vi "Convert Error Cluster to Table.vi"(11 "Error Codes":cluster{i32, string}[](array[cluster])) -> (2 "Code":i32[](array[numeric]), 3 "String":string[](array[string]))   [LabVIEW 2019, in "Ghost Bus Addon System Explorer.lvlib"] (continued)
Explorer</b> window."}, {-307611, "NI VeriStand: The associated NI-XNET database path cannot be found. Please update either the alias or the database path."}, {-307610, "NI VeriStand: The formula contains an invalid function or variable name."}, {-307609, "NI VeriStand: The formula contains an unused variable declaration."}, {-307608, "NI VeriStand: The custom device does not provide a valid source distribution for the target specified. Specify a different target or contact the creator of the custom device for further support."}, {-307607, "NI VeriStand: NI VeriStand could not mutate the system definition file. The system definition file version is different from the official released version of NI VeriStand."}, {-307606, "NI VeriStand: The file does not contain a valid file format."}, {-307605, "NI VeriStand: The requested simulation model could not be found. Navigate to the <b>Model Configuration</b> page in the <b>System Explorer</b> window and choose a different model."}, {-307604, "NI VeriStand: NI VeriStand was unable to mutate the system definition file to the current version."}, {-307603, "NI VeriStand: The requested custom device does not have a main page specified. Contact the creator of the custom device to correct this error."}, {-307602, "NI VeriStand: The GUID could not be found. If the requested page is a custom device, contact the creator of the custom device."}, {-307601, "NI VeriStand: The XML file is invalid according to the XML schema document (XSD)."}, {-307600, "NI VeriStand: The specified VI is broken and cannot run. Open the VI in the LabVIEW development environment for more information."}, {-307562, "NI VeriStand: You cannot use a waveform session reference that you did not first open. Use the NI VeriStand - Open Waveform Session VI to open a waveform session reference."}, {-307561, "NI VeriStand: Cannot write to waveform. Another waveform write session is already open for this waveform reference, and only one writer can access the waveform reference at a time."}, {-307559, "NI VeriStand: The size of an input array does not match the number of waveforms in the streaming session. When you write to a multiple-waveform session, the number of rows in the 2D <B>Data</B> array must match the number of waveforms in the session. When you start a multiple-waveform session, the size of the 1D <B>t0s</B> array must match the number of waveforms in the session."}, {-307557, "NI VeriStand: Custom device cannot perform requested operation because NI VeriStand Engine is shutting down."}, {-307556, "NI VeriStand: Cannot open waveform session because waveform data references are not valid. Use the NI VeriStand - Get Waveform Data Reference VI to generate valid data references with which you can open a waveform session."}, {-307555, "NI VeriStand: Cannot open a waveform session using an empty array of waveform references. Use the NI VeriStand - Get Waveform Data Reference VI to generate valid data references with which you can open a waveform session."}, {-307554, "NI VeriStand: The specified stream condition is not valid for the data type of the waveform. This error might occur if you try to set the streaming condition to be within a range of values for a waveform whose data type is CDB. The in-range streaming condition supports only waveforms whose data type is DBL."}, {-307553, "NI VeriStand: Unexpected waveform data type. This VI requires the specified waveform nodes to be of a specific data type, but the actual data type did not match."}, {-307552, "NI VeriStand: Internal error. An attempt was made to open a 2D waveform read session."}, {-307551, "NI VeriStand: Internal error. The buffered data system failed to find required information in the transaction's variant data."}, {-307550, "NI VeriStand: You have provided an invalid username or password."}, {-307549, "NI VeriStand: Cannot find the wave file that an alarm response is configured to play when the alarm is triggered. Verify that wave files are located at their specified locations. To view and configure this alarm-response setting, open the <B>Project Explorer</B> window, and then double-click an alarm response node underneath <B>Alarm Responses</B> in the tree."}, {-307548, "NI VeriStand: Legacy Stimulus Profile Editor is not supported anymore."}, {-307526, "NI VeriStand: The XML file provided is invalid."}, {-307525, "NI VeriStand: Cannot open selected file. The file was saved in a later version of NI VeriStand."}, {-307512, "NI VeriStand: An unexpected step error has occured."}, {-307511, "NI VeriStand: EESPort with the given name already exists."}, {-307510, "NI VeriStand: Framework with the given name already exists."}, {-307505, "NI VeriStand: The FPGA bitfile has changed since the system definition file was last compiled. Open the system definition file in the <b>System Explorer</b> window and refresh the FPGA configuration file (.fpgaconfig)."}, {-307504, "NI VeriStand: An FPGA argument or parameter is outside the expected range.  This might be a problem with the FPGA configuration file (.fpgaconfig)."}, {-307503, "NI VeriStand: An unknown exception occurred while running the NI-FPGA device. Verify that NI-RIO and the NI VeriStand software are installed correctly on the real-time (RT) target."}, {-307502, "NI VeriStand: An FPGA argument or parameter is invalid. This might be a problem with the FPGA configuration file (.fpgaconfig) or FPGA bitfile. This problem also might be caused by an invalid FPGA target handle."}, {-307501, "NI VeriStand: The specified operation is unable to acquire the memory necessary to execute. To correct this error, increase the amount of memory in the system or reduce the amount of memory that this operation requires. You can reduce the amount of memory required by the operation by uninstalling unneeded components from the real-time (RT) target or by reducing the number of devices, channels, and/or stimulus generators used."}, {307500, "NI VeriStand: The FPGA configuration file (.fpgaconfig) is invalid or contains an error."}, {-1073807360, "VISA:  (Hex 0xBFFF0000) Unknown system error (miscellaneous error)."}, {-1073807346, "VISA:  (Hex 0xBFFF000E) The given session or object reference is invalid."}, {-1073807345, "VISA:  (Hex 0xBFFF000F) Specified type of lock cannot be obtained, or specified operation cannot be performed, because the resource is locked."}, {-1073807344, "VISA:  (Hex 0xBFFF0010) Invalid expression specified for search."}, {-1073807343, "VISA:  (Hex 0xBFFF0011) Insufficient location information or the device or resource is not present in the system."}, {-1073807342, "VISA:  (Hex 0xBFFF0012) Invalid resource reference specified. Parsing error."}, {-1073807341, "VISA:  (Hex 0xBFFF0013) Invalid access mode."}, {-1073807339, "VISA:  (Hex 0xBFFF0015) Timeout expired before operation completed."}, {-1073807338, "VISA:  (Hex 0xBFFF0016) The VISA driver failed to properly close the session or object reference. This might be due to an error freeing internal or OS resources, a failed network connection, or a lower level driver or OS error."}, {-1073807333, "VISA:  (Hex 0xBFFF001B) Specified degree is invalid."}, {-1073807332, "VISA:  (Hex 0xBFFF001C) Specified job identifier is invalid."}, {-1073807331, "VISA:  (Hex 0xBFFF001D) The specified attribute is not defined or supported by the referenced resource."}, {-1073807330, "VISA:  (Hex 0xBFFF001E) The specified state of the attribute is not valid, or is not supported as defined by the resource."}, {-1073807329, "VISA:  (Hex 0xBFFF001F) The specified attribute is read-only."}, {-1073807328, "VISA:  (Hex 0xBFFF0020) The specified type of lock is not supported by this resource."}, {-1073807327, "VISA:  (Hex 0xBFFF0021) The access key to the specified resource is invalid."}, {-1073807322, "VISA:  (Hex 0xBFFF0026) Specified event type is not supported by the resource."}, {-1073807321, "VISA:  (Hex 0xBFFF0027) Invalid mechanism specified."}, {-1073807320, "VISA:  (Hex 0xBFFF0028) A handler was not installed."}, {-1073807319, "VISA:  (Hex 0xBFFF0029) The given handler reference is invalid."}, {-1073807318, "VISA:  (Hex 0xBFFF002A) Specified event context is invalid."}, {-1073807315, "VISA:  (Hex 0xBFFF002D) The event queue for the specified type has overflowed. This is usually due to previous events not having been closed."}, {-1073807313, "VISA:  (Hex 0xBFFF002F) You must be enabled for events of the specified type in order to receive them."}, {-1073807312, "VISA:  (Hex 0xBFFF0030) User abort occurred during transfer."}, {-1073807308, "VISA:  (Hex 0xBFFF0034) Violation of raw write protocol occurred during transfer."}, {-1073807307, "VISA:  (Hex 0xBFFF0035) Violation of raw read protocol occurred during transfer."}, {-1073807306, "VISA:  (Hex 0xBFFF0036) Device reported an output protocol error during transfer."}, {-1073807305, "VISA:  (Hex 0xBFFF0037) Device reported an input protocol error during transfer."}, {-1073807304, "VISA:  (Hex 0xBFFF0038) Bus error occurred during transfer."}, {-1073807303, "VISA:  (Hex 0xBFFF0039) Unable to queue the asynchronous operation because there is already an operation in progress."}, {-1073807302, "VISA:  (Hex 0xBFFF003A) Unable to start operation because setup is invalid (due to attributes being set to an inconsistent state)."}, {-1073807301, "VISA:  (Hex 0xBFFF003B) Unable to queue the asynchronous operation (usually due to the I/O completion event not being enabled or insufficient space in the session's queue)."}, {-1073807300, "VISA:  (Hex 0xBFFF003C) Insufficient system resources to perform necessary memory allocation."}, {-1073807299, "VISA:  (Hex 0xBFFF003D) Invalid buffer mask specified."}, {-1073807298, "VISA:  (Hex 0xBFFF003E) Could not perform operation because of I/O error."}, {-1073807297, "VISA:  (Hex 0xBFFF003F) A format specifier in the format string is invalid."}, {-1073807295, "VISA:  (Hex 0xBFFF0041) A format specifier in the format string is not supported."}, {-1073807294, "VISA:  (Hex 0xBFFF0042) The specified trigger line is currently in use."}, {-1073807293, "VISA:  (Hex 0xBFFF0043) The specified trigger line has not been reserved."}, {-1073807290, "VISA:  (Hex 0xBFFF0046) The specified mode is not supported by this VISA implementation."}, {-1073807286, "VISA:  (Hex 0xBFFF004A) Service request has not been received for the session."}, {-1073807282, "VISA:  (Hex 0xBFFF004E) Invalid address space specified."}, {-1073807279, "VISA:  (Hex 0xBFFF0051) Invalid offset specified."}, {-1073807278, "VISA:  (Hex 0xBFFF0052) Invalid access width specified."}, {-1073807276, "VISA:  (Hex 0xBFFF0054) Specified offset is not accessible from this hardware."}, {-1073807275, "VISA:  (Hex 0xBFFF0055) Cannot support source and destination widths that are different."}, {-1073807273, "VISA:  (Hex 0xBFFF0057) The specified session is not currently mapped."}, {-1073807271, "VISA:  (Hex 0xBFFF0059) A previous response is still pending, causing a multiple query error."}, {-1073807265, "VISA:  (Hex 0xBFFF005F) No listeners condition is detected (both NRFD and NDAC are deasserted)."}, {-1073807264, "VISA:  (Hex 0xBFFF0060) The interface associated with this session is not currently the controller in charge."}, {-1073807263, "VISA:  (Hex 0xBFFF0061) The interface associated with this session is not the system controller."}, {-1073807257, "VISA:  (Hex 0xBFFF0067) The given session or object reference does not support this operation."}, {-1073807256, "VISA:  (Hex 0xBFFF0068) An interrupt is still pending from a previous call."}, {-1073807254, "VISA:  (Hex 0xBFFF006A) A parity error occurred during transfer."}, {-1073807253, "VISA:  (Hex 0xBFFF006B) A framing error occurred during transfer."}, {-1073807252, "VISA:  (Hex 0xBFFF006C) An overrun error occurred during transfer. A character was not read from the hardware before the next character arrived."}, {-1073807250, "VISA:  (Hex 0xBFFF006E) The path from trigSrc to trigDest is not currently mapped."}, {-1073807248, "VISA:  (Hex 0xBFFF0070) The specified offset is not properly aligned for the access width of the operation."}, {-1073807247, "VISA:  (Hex 0xBFFF0071) A specified user buffer is not valid or cannot be accessed for the required size."}, {-1073807246, "VISA:  (Hex 0xBFFF0072) The resource is valid, but VISA cannot currently access it."}, {-1073807242, "VISA:  (Hex 0xBFFF0076) Specified width is not supported by this hardware."}, {-1073807240, "VISA:  (Hex 0xBFFF0078) The value of some parameter (which parameter is not known) is invalid."}, {-1073807239, "VISA:  (Hex 0xBFFF0079) The protocol specified is invalid."}, {-1073807237, "VISA:  (Hex 0xBFFF007B) Invalid size of window specified."}, {-1073807232, "VISA:  (Hex 0xBFFF0080) The specified session currently contains a mapped window."}, {-1073807231, "VISA:  (Hex 0xBFFF0081) The given operation is not implemented."}, {-1073807229, "VISA:  (Hex 0xBFFF0083) Invalid length specified."}, {-1073807215, "VISA:  (Hex 0xBFFF0091) Invalid mode specified."}, {-1073807204, "VISA:  (Hex 0xBFFF009C) The current session did not have a lock on the resource."}, {-1073807203, "VISA:  (Hex 0xBFFF009D) The device does not export any memory."}, {-1073807202, "VISA:  (Hex 0xBFFF009E) VISA or a code library required by VISA could not be located or loaded.  This is usually due to a required driver not being installed on the system."}, {-1073807201, "VISA:  (Hex 0xBFFF009F) The interface cannot generate an interrupt on the requested level or with the requested statusID value."}, {-1073807200, "VISA:  (Hex 0xBFFF00A0) The value specified by the line parameter is invalid."}, {-1073807199, "VISA:  (Hex 0xBFFF00A1) An error occurred while trying to open the specified file. Possible reasons include an invalid path or lack of access rights."}, {-1073807198, "VISA:  (Hex 0xBFFF00A2) An error occurred while performing I/O on the specified file."}, {-1073807197, "VISA:  (Hex 0xBFFF00A3) One of the specified lines, trigSrc or trigDest, is not supported by this VISA implementation, or the combination of lines is not a valid mapping."}, {-1073807196, "VISA:  (Hex 0xBFFF00A4) The specified mechanism is not supported for the given event type."}, {-1073807195, "VISA:  (Hex 0xBFFF00A5) The interface type is valid, but the specified interface number is not configured."}, {-1073807194, "VISA:  (Hex 0xBFFF00A6) The connection for the given session has been lost."}, {-1073807193, "VISA:  (Hex 0xBFFF00A7) The remote machine does not exist or is not accepting any connections. If the NI-VISA server is installed and running on the remote machine, it might have an incompatible version or might be listening on a different port."}, {-1073807192, "VISA:  (Hex 0xBFFF00A8) Access to the resource or remote machine is denied. This is due to lack of sufficient privileges for the current user or machine."}, {-1073807190, "VISA:  (Hex 0xBFFF00AA) A lower level driver reported that this resource corresponds to or is connected to a non-genuine interface. For more information, contact National Instruments support."}, {0, "VISA:  (Hex 0x0) Operation completed successfully."}, {1073676290, "VISA:  (Hex 0x3FFF0002) Specified event is already enabled for at least one of the specified mechanisms."}, {1073676291, "VISA:  (Hex 0x3FFF0003) Specified event is already disabled for at least one of the specified mechanisms."}, {1073676292, "VISA:  (Hex 0x3FFF0004) Operation completed successfully, but queue was already empty."}, {1073676293, "VISA:  (Hex 0x3FFF0005) The specified termination character was read."}, {1073676294, "VISA:  (Hex 0x3FFF0006) The number of bytes transferred is equal to the requested input count. More data might be available."}, {1073676300, "VISA:  (Hex 0x3FFF000C) VISA received more event information of the specified type than the configured queue size could hold."}, {1073676407, "VISA:  (Hex 0x3FFF0077) The specified configuration either does not exist or could not be loaded. VISA-specified defaults will be used."}, {1073676413, "VISA:  (Hex 0x3FFF007D) Session opened successfully, but the device at the specified address is not responding."}, {1073676414, "VISA:  (Hex 0x3FFF007E) The path from trigSrc to trigDest is already mapped."}, {1073676416, "VISA:  (Hex 0x3FFF0080) Wait terminated successfully on receipt of an event notification. There is at least one more event occurrence of the type specified by inEventType available for this session."}, {1073676418, "VISA:  (Hex 0x3FFF0082) The specified object reference is uninitialized."}, {1073676420, "VISA:  (Hex 0x3FFF0084) Although the specified state of the attribute is valid, it is not supported by this resource implementation."}, {1073676421, "VISA:  (Hex 0x3FFF0085) The status code passed to the operation could not be interpreted."}, {1073676424, "VISA:  (Hex 0x3FFF0088) The specified I/O buffer is not supported."}, {1073676440, "VISA:  (Hex 0x3FFF0098) Event handled successfully. Do not invoke any other handlers on this session for this event."}, {1073676441, "VISA:  (Hex 0x3FFF0099) Operation completed successfully, and this session has nested shared locks."}, {1073676442, "VISA:  (Hex 0x3FFF009A) Operation completed successfully, and this session has nested exclusive locks."}, {1073676443, "VISA:  (Hex 0x3FFF009B) Operation completed successfully, but the operation was actually synchronous rather than asynchronous."}, {1073676457, "VISA:  (Hex 0x3FFF00A9) The operation succeeded, but a lower level driver did not implement the extended functionality."}, {-2147483638, "LabVIEW: (Hex 0x8000000A) The data necessary to complete this operation is not yet available."}, {-2147467263, "LabVIEW: (Hex 0x80004001) Not implemented."}, {-2147467262, "LabVIEW: (Hex 0x80004002) No such interface supported."}, {-2147467261, "LabVIEW: (Hex 0x80004003) Invalid pointer."}, {-2147467260, "LabVIEW: (Hex 0x80004004) Operation aborted."}, {-2147467259, "LabVIEW: (Hex 0x80004005) Unspecified error."}, {-2147418113, "LabVIEW: (Hex 0x8000FFFF) Catastrophic failure."}, {-2147024891, "LabVIEW: (Hex 0x80070005) Access denied. This error can occur if you attempt to write a single writer shared variable that is already connected to a subscriber with write access. Ensure that you connect only one target with write access to this shared variable at a time."}, {-2147024890, "LabVIEW: (Hex 0x80070006) Invalid handle."}, {-2147024882, "LabVIEW: (Hex 0x8007000E) Ran out of memory."}, {-2147024809, "LabVIEW: (Hex 0x80070057) One or more arguments are invalid."}, {-2132869120, "LabVIEW: (Hex 0x80DF0000) The assembly you are deploying is bad."}, {-2132869119, "LabVIEW: (Hex 0x80DF0001) The assembly handler does not support the sent command."}, {-2132869118, "LabVIEW: (Hex 0x80DF0002) A file I/O error occurred."}, {-2132869117, "LabVIEW: (Hex 0x80DF0003) The resource you are deploying is bad."}, {-2132869116, "LabVIEW: (Hex 0x80DF0004) The item cannot read the assembly."}, {-2132869115, "LabVIEW: (Hex 0x80DF0005) The item cannot create the assembly handler."}, {-2132869114, "LabVIEW: (Hex 0x80DF0006) A module cannot load."}, {-2132869113, "LabVIEW: (Hex 0x80DF0007) The item encountered an invalid pointer argument."}, {-2132869112, "LabVIEW: (Hex 0x80DF0008) The item cannot be found."}, {-2132869111, "LabVIEW: (Hex 0x80DF0009) The item is out of memory."}, {-2132869110, "LabVIEW: (Hex 0x80DF000A) A communication error between the host and target occurred."}, {-2132869109, "LabVIEW: (Hex 0x80DF000B) The system is in a bad state."}, {-2132869108, "LabVIEW: (Hex 0x80DF000C) The deploy header is bad."}, {-2132869107, "LabVIEW: (Hex 0x80DF000D) An unknown error occurred during deployment."}, {-2132869106, "LabVIEW: (Hex 0x80DF000E) An XML parsing error occurred."}, {-2132869105, "LabVIEW: (Hex 0x80DF000F) The deployment command failed."}, {-2132869104, "LabVIEW: (Hex 0x80DF0010) The current deployment operation has a missing dependency."}, {-2132869103, "LabVIEW: (Hex 0x80DF0011) The item encountered an invalid argument."}, {-2132869102, "LabVIEW: (Hex 0x80DF0012) The specified file cannot be found."}, {-2132869101, "LabVIEW: (Hex 0x80DF0013) The deployment operation caused a rollback operation, and the rollback operation failed."}, {-2132869100, "LabVIEW: (Hex 0x80DF0014) Logging an entry to the rollback log causes an error."}, {-2132869099, "LabVIEW: (Hex 0x80DF0015) A deployment transaction is in progress."}, {-2132869098, "LabVIEW: (Hex 0x80DF0016) A deployment transaction has not started."}, {-2132869096, "LabVIEW: (Hex 0x80DF0018) The deployment operation causes a rollback operation."}, {-2132869095, "LabVIEW: (Hex 0x80DF0019) The deployment connection timed out."}, {-2132869094, "LabVIEW: (Hex 0x80DF001A) The current transaction has no items to process."}, {-2132869093, "LabVIEW: (Hex 0x80DF001B) The current state does not allow the deployment operation."}, {-2132869092, "LabVIEW: (Hex 0x80DF001C) No items are left to deploy."}, {-2132869091, "LabVIEW: (Hex 0x80DF001D) No items are left to undeploy."}, {-2132869090, "LabVIEW: (Hex 0x80DF001E) The deployment plug-in for this item cannot be found. Verify the proper software is installed."}, {-2132869089, "LabVIEW: (Hex 0x80DF001F) An instance of the target-side deployment endpoint already exists."}, {-2132869088, "LabVIEW: (Hex 0x80DF0020) This item cannot upload because another item with the same name exists in the project."}, {-2067353911, "LabVIEW: (Hex 0x84C6AEC9) The data type of a process variable in the EPICS Client I/O server does not match the data type of the corresponding process variable in the IOC."}, {-2067353910, "LabVIEW: (Hex 0x84C6AECA) The connection to the IOC was lost due to a network failure or an IOC error."}, {-2067353909, "LabVIEW: (Hex 0x84C6AECB) The EPICS Server I/O Server cannot be deployed because one or more PV source variables do not exist. Open the configuration dialog to check and correct broken source variables."}, {-2000000013, "LabVIEW: (Hex 0x88CA6BF3) Input Sprockets Failure. The Mac Input Sprockets Toolkit is not properly installed on the machine."}, {-2000000012, "LabVIEW: (Hex 0x88CA6BF4) Close failure. Make sure the device is currently open."}, {-2000000011, "LabVIEW: (Hex 0x88CA6BF5) Read failure. Failed to read the device."}, {-2000000010, "LabVIEW: (Hex 0x88CA6BF6) The device ID being passed in is incorrect. Please connect the device ID parameter from the Initialize VI to the input parameter of the Close Input Device VI."}, {-2000000009, "LabVIEW: (Hex 0x88CA6BF7) The operation cannot be performed while the device is being acquired."}, {-2000000008, "LabVIEW: (Hex 0x88CA6BF8) Invalid device index. Please check to see if the device is attached correctly. Please verify that the device index you passed in to the Initialize Device VI is correct."}, {-2000000007, "LabVIEW: (Hex 0x88CA6BF9) Data is not yet available."}, {-2000000006, "LabVIEW: (Hex 0x88CA6BFA) The operation cannot be performed unless the device is acquired."}, {-2000000005, "LabVIEW: (Hex 0x88CA6BFB) Access to the input device has been lost. You must reacquire access to the input device."}, {-2000000004, "LabVIEW: (Hex 0x88CA6BFC) This object has not been initialized."}, {-2000000003, "LabVIEW: (Hex 0x88CA6BFD) The DirectInput subsystem could not allocate sufficient memory to complete the call. This value is equal to the E_OUTOFMEMORY standard COM return value."}, {-2000000002, "LabVIEW: (Hex 0x88CA6BFE) The application requires a newer version of DirectInput."}, {-2000000001, "LabVIEW: (Hex 0x88CA6BFF) An invalid parameter was passed to the returning function, or the object was not in a state that permitted the function to be called. This value is equal to the E_INVALIDARG standard COM return value."}, {-2000000000, "LabVIEW: (Hex 0x88CA6C00) The application was written for an unsupported prerelease version of DirectInput."}, {-1967390719, "LabVIEW: (Hex 0x8ABC0001) Packet is too short or too long."}, {-1967390717, "LabVIEW: (Hex 0x8ABC0003) Command not allowed in this particular context."}, {-1967390716, "LabVIEW: (Hex 0x8ABC0004) Duplicate item already exists."}, {-1967390715, "LabVIEW: (Hex 0x8ABC0005) Item not found."}, {-1967390714, "LabVIEW: (Hex 0x8ABC0006) Interface object not valid."}, {-1967390713, "LabVIEW: (Hex 0x8ABC0007) Target of Modify() already has an input connection."}, {-1967390712, "LabVIEW: (Hex 0x8ABC0008) Cannot resolve name to a network address."}, {-1967390711, "LabVIEW: (Hex 0x8ABC0009) Network operation timed out."}, {-1967390704, "LabVIEW: (Hex 0x8ABC0010) Socket has been disconnected by its peer."}, {-1967390703, "LabVIEW: (Hex 0x8ABC0011) Could not resolve service to a port address."}, {-1967390702, "LabVIEW: (Hex 0x8ABC0012) Timed out while trying to connect to peer."}, {-1967390701, "LabVIEW: (Hex 0x8ABC0013) Socket startup (WSAStartup) failed."}, {-1967390687, "LabVIEW: (Hex 0x8ABC0021) The URL is to short to contain the minimum amount of information or the pointer is invalid."}, {-1967390686, "LabVIEW: (Hex 0x8ABC0022) Computer name is not present in the URL."}, {-1967390685, "LabVIEW: (Hex 0x8ABC0023) Computer name starts with a non-alphabetic character."}, {-1967390684, "LabVIEW: (Hex 0x8ABC0024) Computer name contains an invalid character."}, {-1967390683, "LabVIEW: (Hex 0x8ABC0025) Process name is not present in the URL."}, {-1967390682, "LabVIEW: (Hex 0x8ABC0026) Process name contains an invalid character."}, {-1967390681, "LabVIEW: (Hex 0x8ABC0027) Point or tag name is not present in the URL."}, {-1967390680, "LabVIEW: (Hex 0x8ABC0028) Point or tag name contains an invalid character."}, {-1967390679, "LabVIEW: (Hex 0x8ABC0029) URL is not properly formatted: not enough '\\' characters at the beginning."}, {-1967390672, "LabVIEW: (Hex 0x8ABC0030) Empty component in point or tag name."}, {-1967390671, "LabVIEW: (Hex 0x8ABC0031) Invalid update rate."}, {-1967390670, "LabVIEW: (Hex 0x8ABC0032) Invalid deadband."}, {-1967390669, "LabVIEW: (Hex 0x8ABC0033) Key conflict for map collection on insert."}, {-1967390668, "LabVIEW: (Hex 0x8ABC0034) Thread initiation failed."}, {-1967390667, "LabVIEW: (Hex 0x8ABC0035) Process manager server is down."}, {-1967390666, "LabVIEW: (Hex 0x8ABC0036) Time stamp at RealTimeTQ not ready."}, {-1967390655, "LabVIEW: (Hex 0x8ABC0041) Object environment server has already shut down."}, {-1967390638, "LabVIEW: (Hex 0x8ABC0052) Item not found."}, {-1967390623, "LabVIEW: (Hex 0x8ABC0061) Attempted to resolve an incomplete URL."}, {-1967390622, "LabVIEW: (Hex 0x8ABC0062) Attempted to resolve an unrecognized URL type."}, {-1967390621, "LabVIEW: (Hex 0x8ABC0063) Process server has already shut down."}, {-1967390620, "LabVIEW: (Hex 0x8ABC0064) Access request denied."}, {-1967390591, "LabVIEW: (Hex 0x8ABC0081) Unable to resolve the host name."}, {-1967390590, "LabVIEW: (Hex 0x8ABC0082) Unable to resolve the IP address returned from gethostbyname()."}, {-1967390575, "LabVIEW: (Hex 0x8ABC0091) Unrecognized attribute name."}, {-1967390574, "LabVIEW: (Hex 0x8ABC0092) Invalid attribute value."}, {-1967390573, "LabVIEW: (Hex 0x8ABC0093) Failed to get or set attribute."}, {-1967390464, "LabVIEW: (Hex 0x8ABC0100) URL does not start with two slashes."}, {-1967390463, "LabVIEW: (Hex 0x8ABC0101) URL starts with more than two slashes."}, {-1967390462, "LabVIEW: (Hex 0x8ABC0102) URL contains two consecutive delimiters."}, {-1967390461, "LabVIEW: (Hex 0x8ABC0103) URL contains a bad machine name."}, {-1967390460, "LabVIEW: (Hex 0x8ABC0104) Unbalanced quotation marks in URL."}, {-1967345152, "LabVIEW: (Hex 0x8ABCB200) Invalid refnum."}, {-1967345151, "LabVIEW: (Hex 0x8ABCB201) Invalid property code."}, {-1967345150, "LabVIEW: (Hex 0x8ABCB202) Invalid privilege ID."}, {-1967345149, "LabVIEW: (Hex 0x8ABCB203) Invalid access type."}, {-1967345148, "LabVIEW: (Hex 0x8ABCB204) Invalid argument."}, {-1967345147, "LabVIEW: (Hex 0x8ABCB205) Entry not found."}, {-1950679041, "LabVIEW: (Hex 0x8BBAFFFF) The prototype of a shared variable whose data type is custom cannot be an empty variant."}, {-1950679040, "LabVIEW: (Hex 0x8BBB0000) The value from this shared variable might not be the most current value from the data source."}, {-1950679039, "LabVIEW: (Hex 0x8BBB0001) Sensor failure"}, {-1950679038, "LabVIEW: (Hex 0x8BBB0002) General device error response."}, {-1950679037, "LabVIEW: (Hex 0x8BBB0003) The shared variable specified in the binding URL does not exist in the process. Ensure that all shared variables are deployed and the variable identifier URL is correct."}, {-1950679036, "LabVIEW: (Hex 0x8BBB0004) General communications failure."}, {-1950679035, "LabVIEW: (Hex 0x8BBB0005) Unable to locate the shared variable in the Shared Variable Engine (SVE). Deployment of this shared variable may have failed, the SVE has not started, or the SVE is too busy to respond to this request."}, {-1950679034, "LabVIEW: (Hex 0x8BBB0006) The shared variable has no value."}, {-1950679033, "LabVIEW: (Hex 0x8BBB0007) The shared variable is inactive."}, {-1950679032, "LabVIEW: (Hex 0x8BBB0008) Sensor inaccurate"}, {-1950679031, "LabVIEW: (Hex 0x8BBB0009) Engineering unit limits exceeded."}, {-1950679030, "LabVIEW: (Hex 0x8BBB000A) Unspecified error"}, {-1950679029, "LabVIEW: (Hex 0x8BBB000B) Math error"}, {-1950679028, "LabVIEW: (Hex 0x8BBB000C) Communications link failure"}, {-1950679027, "LabVIEW: (Hex 0x8BBB000D) NI-PSP has not connected to the server yet"}, {-1950679026, "LabVIEW: (Hex 0x8BBB000E) DNS lookup failed for the server."}, {-1950679025, "LabVIEW: (Hex 0x8BBB000F) The server is not reachable."}, {-1950679024, "LabVIEW: (Hex 0x8BBB0010) Service lookup failed for the server."}, {-1950679023, "LabVIEW: (Hex 0x8BBB0011) The process specified in the binding URL does not exist. Ensure that all shared variables are deployed and the variable identifier URL is correct."}, {-1950679022, "LabVIEW: (Hex 0x8BBB0012) The process was not found or is not responding."}, {-1950679021, "LabVIEW: (Hex 0x8BBB0013) Failed to resolve URL for this shared variable."}, {-1950679020, "LabVIEW: (Hex 0x8BBB0014) Unable to access the shared variable. This error can occur if you attempt to read from a write-only variable or write to a read-only variable, or if you do not have permission to access the variable."}, {-1950679019, "LabVIEW: (Hex 0x8BBB0015) Subscribe failed. This error can occur when a client attempts to connect to a host using Logos, when the host only supports LogosXT."}, {-1950679018, "LabVIEW: (Hex 0x8BBB0016) Invalid URL for this shared variable."}, {-1950679017, "LabVIEW: (Hex 0x8BBB0017) Invalid combination of feature packs"}, {-1950679016, "LabVIEW: (Hex 0x8BBB0018) Invalid float value."}, {-1950679015, "LabVIEW: (Hex 0x8BBB0019) Invalid Boolean value."}, {-1950679014, "LabVIEW: (Hex 0x8BBB001A) Value attribute not found."}, {-1950679013, "LabVIEW: (Hex 0x8BBB001B) Invalid access type."}, {-1950679012, "LabVIEW: (Hex 0x8BBB001C) Missing access type."}, {-1950679011, "LabVIEW: (Hex 0x8BBB001D) Invalid URL syntax."}, {-1950679010, "LabVIEW: (Hex 0x8BBB001E) Shared variable is bound but the path or URL is not specified."}, {-1950679009, "LabVIEW: (Hex 0x8BBB001F) A path and URL are both specified."}, {-1950679008, "LabVIEW: (Hex 0x8BBB0020) Invalid value for the <b>Enable Aliasing</b> option."}, {-1950679007, "LabVIEW: (Hex 0x8BBB0021) A value is missing for the Enable Aliasing option."}, {-1950679006, "LabVIEW: (Hex 0x8BBB0022) Invalid value for Single Writer option."}, {-1950679005, "LabVIEW: (Hex 0x8BBB0023) You must select a name for the shared variable."}, {-1950679004, "LabVIEW: (Hex 0x8BBB0024) Two var type feature packs are selected"}, {-1950679003, "LabVIEW: (Hex 0x8BBB0025) No var type feature pack is selected"}, {-1950679002, "LabVIEW: (Hex 0x8BBB0026) Var type feature packs must be required"}, {-1950679001, "LabVIEW: (Hex 0x8BBB0027) Buffer size must be greater than 1."}, {-1950679000, "LabVIEW: (Hex 0x8BBB0028) Array length must be greater than or equal to 2."}, {-1950678999, "LabVIEW: (Hex 0x8BBB0029) Data points in waveform must be greater than or equal to 1."}, {-1950678998, "LabVIEW: (Hex 0x8BBB002A) Global variables can only be accessed from the local machine."}, {-1950678997, "LabVIEW: (Hex 0x8BBB002B) You cannot use a Variable Node of this type on this target."}, {-1950678996, "LabVIEW: (Hex 0x8BBB002C) The variable configuration is invalid.  Edit the variable properties to correct the configuration."}, {-1950678995, "LabVIEW: (Hex 0x8BBB002D) Variable has undefined data type."}, {-1950678994, "LabVIEW: (Hex 0x8BBB002E) Variable has invalid data type."}, {-1950678993, "LabVIEW: (Hex 0x8BBB002F) The Raw Full Scale value must be greater than the Raw Zero Scale value."}, {-1950678992, "LabVIEW: (Hex 0x8BBB0030) The Raw Scale and/or Engineering Scale is invalid."}, {-1950678991, "LabVIEW: (Hex 0x8BBB0031) The Engineering Full Scale value should not be equal to Engineering Zero Scale value."}, {-1950678990, "LabVIEW: (Hex 0x8BBB0032) Scaling type attribute not specified."}, {-1950678989, "LabVIEW: (Hex 0x8BBB0033) Scaling ranges not fully specified."}, {-1950678988, "LabVIEW: (Hex 0x8BBB0034) The number of arrays, elements, and points per waveform must be greater than or equal to 1."}, {-1950678987, "LabVIEW: (Hex 0x8BBB0035) This piece of configuration does not exist for this type of variable."}, {-1950678986, "LabVIEW: (Hex 0x8BBB0036) Unspecified shared variable error."}, {-1950678985, "LabVIEW: (Hex 0x8BBB0037) Invalid variable name. The name of a variable cannot start with a single quote ('), start or end with a space, or contain a backslash, forward slash, or any of the following backslash '\\' codes: \\r \\n \\t \\b \\s."}, {-1950678984, "LabVIEW: (Hex 0x8BBB0038) Variable names can have a maximum of 255 characters."}, {-1950678983, "LabVIEW: (Hex 0x8BBB0039) The array sizes in the network buffer must be greater than or equal to the array sizes in the real-time FIFO buffer. The waveform sizes in the network buffer must be greater than or equal to the waveform sizes in the real-time FIFO buffer."}, {-1950678982, "LabVIEW: (Hex 0x8BBB003A) The shared variable client-side read buffer is full."}, {-1950678981, "LabVIEW: (Hex 0x8BBB003B) The shared variable client-side read buffer overflowed."}, {-1950678980, "LabVIEW: (Hex 0x8BBB003C) The shared variable server-side write buffer is full."}, {-1950678979, "LabVIEW: (Hex 0x8BBB003D) The shared variable server-side write buffer overflowed."}, {-1950678978, "LabVIEW: (Hex 0x8BBB003E) The project that contains the project library you want to add a shared variable to must be open."}, {-1950678977, "LabVIEW: (Hex 0x8BBB003F) Unable to deploy the library because the name is reserved. You cannot deploy a library named \"System\", \"LV\", or \"FP\". You also cannot deploy a library with a name that starts with \"NI_\"."}, {-1950678976, "LabVIEW: (Hex 0x8BBB0040) Attempted to load, replace, or remove a configuration from a different source. Your configuration might conflict with the NI Scan Engine configuration."}, {-1950678975, "LabVIEW: (Hex 0x8BBB0041) Invalid Integer value."}, {-1950678974, "LabVIEW: (Hex 0x8BBB0042) Invalid Logging String Format"}, {-1950678972, "LabVIEW: (Hex 0x8BBB0044) LabVIEW failed to load Logos."}, {-1950678971, "LabVIEW: (Hex 0x8BBB0045) LabVIEW could not resolve the machine alias for this Shared Variable and is using a cached IP Address instead."}, {-1950678970, "LabVIEW: (Hex 0x8BBB0046) Failed to load rtvarsup, which is required for Shared Variables with the Real-Time FIFO enabled."}, {-1950678969, "LabVIEW: (Hex 0x8BBB0047) Failed to load rtvarnet, which is required for Network-Published Shared Variables with the Real-Time FIFO enabled."}, {-1950678968, "LabVIEW: (Hex 0x8BBB0048) Failed to load nitaglv, which is required for Network-Published Shared Variables."}, {-1950678967, "LabVIEW: (Hex 0x8BBB0049) Aliasee is missing."}, {-1950678966, "LabVIEW: (Hex 0x8BBB004A) Cannot access I/O variables in Direct mode remotely."}, {-1950678965, "LabVIEW: (Hex 0x8BBB004B) The value read is of a data type that cannot be converted to the data type of this Shared Variable node."}, {-1950678964, "LabVIEW: (Hex 0x8BBB004C) Failed to load NI Scan Engine software required for I/O Variable access.  If you are hosting I/O variables on an RT target, ensure that the NI Scan Engine is installed on the RT target. If you are hosting I/O variables on Windows, you must install a Windows I/O driver, such as DeviceNet, that includes NI Scan Engine support. If you are hosting I/O variables in a Windows VI, the VI must be part of an open LabVIEW project. If you are hosting I/O variables in a Windows-built application, the application must be configured to include hardware configuration."}, {-1950678963, "LabVIEW: (Hex 0x8BBB004D) Unable to open the variable connection. A connection to the specified variable is already open using a different data type."}, {-1950678962, "LabVIEW: (Hex 0x8BBB004E) The specified variable does not support the specified read, write, or open operation."}, {-1950678961, "LabVIEW: (Hex 0x8BBB004F) The connection to the variable has been closed."}, {-1950678960, "LabVIEW: (Hex 0x8BBB0050) The specified variable connection is not configured to read timestamps."}, {-1950678959, "LabVIEW: (Hex 0x8BBB0051) The specified I/O Variable is configured with a timeout, but timeouts are not supported when accessing an I/O variable locally."}, {-1950678958, "LabVIEW: (Hex 0x8BBB0052) This property can be called only on an I/O alias."}, {-1950678957, "LabVIEW: (Hex 0x8BBB0053) This property can be called only on an I/O variable."}, {-1950678956, "LabVIEW: (Hex 0x8BBB0054) The property cannot be set when the variable is reserved."}, {-1950678955, "LabVIEW: (Hex 0x8BBB0055) Invalid URL. The URL cannot contain # or ? characters."}, {-1950678954, "LabVIEW: (Hex 0x8BBB0056) The string for the Variable Engine or protocol portion of the URL is invalid."}, {-1950678953, "LabVIEW: (Hex 0x8BBB0057) The URL is invalid."}, {-1950678952, "LabVIEW: (Hex 0x8BBB0058) The URL is invalid.  The URL contains the User Information subcomponent within the Authority which isn't supported by this scheme.  If you included the \"@\" character as part of the Authority and didn't intend for it to signify the User Information field, replace the \"@\" character with its percent encode UTF-8 equivalent form of \"%40\"."}, {-1950678951, "LabVIEW: (Hex 0x8BBB0059) The host name specified in the URL is invalid.  It contains one or more of the characters \":/?#[]@\" which are illegal to use in their decoded form.  If the host name contains one of these characters, replace it with its percent encoded UTF-8 equivalent form.  For example, to specify the host name \"My Machine?\" you must use the string \"My Machine%3F\"."}, {-1950678950, "LabVIEW: (Hex 0x8BBB005A) The port specified in the Authority component of the URL is invalid.  The port must consist of only numeric characters."}, {-1950678949, "LabVIEW: (Hex 0x8BBB005B) The URL contains one or more unsupported path segments.  Path segments of the form \"/./\", \"/../\", and empty path segments \"//\" are not supported."}, {-1950678948, "LabVIEW: (Hex 0x8BBB005C) The path in the URL is invalid."}, {-1950678947, "LabVIEW: (Hex 0x8BBB005D) The specified URL is invalid.  The URL specifies a host name that includes a port.  However, ports are not supported by the specified variable engine."}, {-1950678946, "LabVIEW: (Hex 0x8BBB005E) The specified URL contains a relative path reference, but LabVIEW does not support relative paths in Variable URLs. To correct the problem, use absolute path references instead of relative references. Variable URLs must take one of the following three forms: (1) [Variable Engine]://[Host Name]/[Container Name]/[Variable Name] or (2) //[Host Name]/[Container Name]/[Variable Name] or (3) /[Container Name]/[Variable Name]."}, {-1950678945, "LabVIEW: (Hex 0x8BBB005F) The host name specified in the variable identifier URL does not correspond to the local host, but the specified variable engine URL only supports an operation on the local host. You cannot perform the specified operation on a remotely hosted variable or stream endpoint. Use the PSP Variable Engine URL (ni.var.psp) to read or write a network-published I/O variable or I/O alias remotely."}, {-1950678944, "LabVIEW: (Hex 0x8BBB0060) The Class Identifier property of the variable object specified in the variable identifier URL is incompatible with the refnum configuration. The class of the variable object is not equivalent to or does not derive from the class you configured for the refnum. This error might occur if you try to reference a <b>Variable</b> object, but the specified variable identifier URL does not reference a <b>Variable</b>."}, {-1950678943, "LabVIEW: (Hex 0x8BBB0061) Timed out while attempting to open a connection to the variable."}, {-1950678942, "LabVIEW: (Hex 0x8BBB0062) Scaling coerce attribute not specified."}, {-1950678941, "LabVIEW: (Hex 0x8BBB0063) An empty string is not a valid URL.  If you want to reference the root container within a variable engine, you need to specify the path explicitly using one of the following URL formats: \"[Variable Engine]://[Host Name]\", \"[Variable Engine]:\", or \"/\"."}, {-1950678940, "LabVIEW: (Hex 0x8BBB0064) The remote configuration web service is not installed on the host specified in the URL."}, {-1950678939, "LabVIEW: (Hex 0x8BBB0065) The version of the remote configuration web service installed on the host specified in the URL is not compatible with this version of LabVIEW."}, {-1950678938, "LabVIEW: (Hex 0x8BBB0066) The NI Vision software is not installed.  This datatype can only be used when NI Vision is installed."}, {-1950678937, "LabVIEW: (Hex 0x8BBB0067) An attempt was made to read or write a property that is only valid for readable variable objects."}, {-1950678936, "LabVIEW: (Hex 0x8BBB0068) The specified buffer size is invalid.  Valid values are zero and sizes greater than two.  A buffer size of zero will disable buffering and cause the connection to maintain only the latest value."}, {-1950678935, "LabVIEW: (Hex 0x8BBB0069) The scheme specified in the URL is not supported."}, {-1950678934, "LabVIEW: (Hex 0x8BBB006A) Requires an open variable connection to read or write the specified property."}, {-1074003967, "LabVIEW: (Hex 0xBFFC0001) Parameter 1 is out of range."}, {-1074003966, "LabVIEW: (Hex 0xBFFC0002) Parameter 2 is out of range."}, {-1074003965, "LabVIEW: (Hex 0xBFFC0003) Parameter 3 is out of range."}, {-1074003964, "LabVIEW: (Hex 0xBFFC0004) Parameter 4 is out of range."}, {-1074003963, "LabVIEW: (Hex 0xBFFC0005) Parameter 5 is out of range."}, {-1074003962, "LabVIEW: (Hex 0xBFFC0006) Parameter 6 is out of range."}, {-1074003961, "LabVIEW: (Hex 0xBFFC0007) Parameter 7 is out of range."}, {-1074003960, "LabVIEW: (Hex 0xBFFC0008) Parameter 8 is out of range."}, {-1074003952, "LabVIEW: (Hex 0xBFFC0010) Error interpreting instrument response"}, {-1074003951, "LabVIEW: (Hex 0xBFFC0011) Identification query failed."}, {-1074003950, "LabVIEW: (Hex 0xBFFC0012) Error interpreting the instrument's response."}, {-1074000001, "LabVIEW: (Hex 0xBFFC0F7F) Instrument self-test failure."}, {-1074000000, "LabVIEW: (Hex 0xBFFC0F80) Instrument error query failure."}, {-1073807202, "LabVIEW: (Hex 0xBFFF009E) VISA or a code library required by VISA could not be located or loaded.  This is usually due to a required driver not being installed on the system."}, {-389122, "LabVIEW: (Hex 0xFFFA0FFE) The target device does not have any response. Possible reason: the target device is not present on the network."}, {-389121, "LabVIEW: (Hex 0xFFFA0FFF) The gateway is unable to allocate an internal communication path from the input port to the output port for processing the request. Possible reason: the gateway is either misconfigured or overloaded."}, {-389118, "LabVIEW: (Hex 0xFFFA1002) An extended file area failed to pass a consistency check. You can use the Modbus master to retry the connection, but the Modbus slave may require certain service."}, {-389116, "LabVIEW: (Hex 0xFFFA1004) The Modbus slave is busy. Use the Modbus master to retransmit data at a later time."}, {-389115, "LabVIEW: (Hex 0xFFFA1005) The Modbus slave is processing the request and may spend a long time processing this request."}, {-389114, "LabVIEW: (Hex 0xFFFA1006) An unrecoverable error occurred while the server was attempting to perform the requested action."}, {-389113, "LabVIEW: (Hex 0xFFFA1007) A value contained in the query data field is invalid for the Modbus slave."}, {-389112, "LabVIEW: (Hex 0xFFFA1008) The Modbus slave does not accept the data address contained in the query."}, {-389111, "LabVIEW: (Hex 0xFFFA1009) The Modbus slave does not accept the function code contained in the query."}, {-389107, "LabVIEW: (Hex 0xFFFA100D) The Modbus master does not use a serial protocol and cannot perform the action that you requested. Ensure that you use a serial Modbus master to perform this action."}, {-389106, "LabVIEW: (Hex 0xFFFA100E) The current Modbus slave cannot perform the operation you wanted to perform, because this slave is not a TCP Modbus slave."}, {-389105, "LabVIEW: (Hex 0xFFFA100F) The Modbus slave daemon, also known as background process, failed to launch. Contact National Instruments for technical support."}, {-389104, "LabVIEW: (Hex 0xFFFA1010) The object that you write exceeds 244 bytes in length."}, {-389103, "LabVIEW: (Hex 0xFFFA1011) The object that you specified does not exist in the Modbus slave. Ensure that you specify an object that exists in the Modbus slave. Contact National Instruments for technical support."}, {-389102, "LabVIEW: (Hex 0xFFFA1012) The data that the Modbus slave returned did not match the data that the Modbus master sent for the operation you want to perform. Contact National Instruments for technical support."}, {-389101, "LabVIEW: (Hex 0xFFFA1013) The returned Modbus Encapsulated Interface type was not 0x0E (14). This type is required for the operation you want to perform. Possible reasons: the Modbus slave does not have a device identification; the Modbus slave does not support read operations on its device identification."}, {-389100, "LabVIEW: (Hex 0xFFFA1014) The returned function code does not match the function code in the requested data. Contact National Instruments for technical support."}, {-375800, "LabVIEW: (Hex 0xFFFA4408) You cannot append variable-sized records, such as strings, handles, or arrays, to a datalog file that is larger than 4GB."}, {-375704, "LabVIEW: (Hex 0xFFFA4468) Invalid channel index."}, {-375703, "LabVIEW: (Hex 0xFFFA4469) Data type mismatch."}, {-375702, "LabVIEW: (Hex 0xFFFA446A) Invalid value index."}, {-375701, "LabVIEW: (Hex 0xFFFA446B) The Excel file is not generated by LabVIEW."}, {-375628, "LabVIEW: (Hex 0xFFFA44B4) Invalid ISO3166 code."}, {-375627, "LabVIEW: (Hex 0xFFFA44B5) Invalid transaction."}, {-375626, "LabVIEW: (Hex 0xFFFA44B6) Operation is not permitted because a transaction was not started."}, {-375625, "LabVIEW: (Hex 0xFFFA44B7) Index out of range."}, {-375624, "LabVIEW: (Hex 0xFFFA44B8) Unexpected OS error."}, {-375623, "LabVIEW: (Hex 0xFFFA44B9) The scan operation took too long."}, {-375622, "LabVIEW: (Hex 0xFFFA44BA) WPA communication error."}, {-375621, "LabVIEW: (Hex 0xFFFA44BB) DBus communication error."}, {-375571, "LabVIEW: (Hex 0xFFFA44ED) Unable to complete the current EtherCAT request."}, {-375570, "LabVIEW: (Hex 0xFFFA44EE) Unable to get the current device configuration."}, {-375569, "LabVIEW: (Hex 0xFFFA44EF) Unable to set the primary device."}, {-375568, "LabVIEW: (Hex 0xFFFA44F0) Unable to get a valid dns address."}, {-375567, "LabVIEW: (Hex 0xFFFA44F1) Unable to get valid gateway address."}, {-375566, "LabVIEW: (Hex 0xFFFA44F2) Unable to get valid IP address."}, {-375565, "LabVIEW: (Hex 0xFFFA44F3) Unable to set current IP configuration"}, {-375564, "LabVIEW: (Hex 0xFFFA44F4) Unable to complete current request."}, {-375563, "LabVIEW: (Hex 0xFFFA44F5) Invalid input parameter."}, {-375562, "LabVIEW: (Hex 0xFFFA44F6) The buffer provided was too small."}, {-375561, "LabVIEW: (Hex 0xFFFA44F7) Operation invalid because IP address index is out of range."}, {-375560, "LabVIEW: (Hex 0xFFFA44F8) Operation not permitted because device index is out of range."}, {-375533, "LabVIEW: (Hex 0xFFFA4513) Unable to set option \"Halt on IP failure\"."}, {-375532, "LabVIEW: (Hex 0xFFFA4514) Unable to get the disk space information."}, {-375531, "LabVIEW: (Hex 0xFFFA4515) Unable to get the target's class."}, {-375530, "LabVIEW: (Hex 0xFFFA4516) Unable to get the target's firmware version."}, {-375529, "LabVIEW: (Hex 0xFFFA4517) Unable to get the target's device description."}, {-375528, "LabVIEW: (Hex 0xFFFA4518) Unable to set user comment."}, {-375527, "LabVIEW: (Hex 0xFFFA4519) Unable to get the target's hostname."}, {-375526, "LabVIEW: (Hex 0xFFFA451A) Unable to set the current hostname."}, {-375525, "LabVIEW: (Hex 0xFFFA451B) Unable to get daylight savings rule."}, {-375524, "LabVIEW: (Hex 0xFFFA451C) Unable to set current daylight savings rule."}, {-375523, "LabVIEW: (Hex 0xFFFA451D) Unable to validate the current timezone."}, {-375522, "LabVIEW: (Hex 0xFFFA451E) Unable to get the current timezone."}, {-375521, "LabVIEW: (Hex 0xFFFA451F) Unable to set current timezone."}, {-375520, "LabVIEW: (Hex 0xFFFA4520) Unable to set current language."}, {-375502, "LabVIEW: (Hex 0xFFFA4532) The current operation is not implemented."}, {-375501, "LabVIEW: (Hex 0xFFFA4533) Unexpected error while executing the current operation."}, {-375500, "LabVIEW: (Hex 0xFFFA4534) There isn't enough memory to complete the current operation."}, {-375324, "LabVIEW: (Hex 0xFFFA45E4) An unknown or unexpected communication fault occurred while attempting to read data from or write data to a device."}, {-375323, "LabVIEW: (Hex 0xFFFA45E5) No transfer is in progress because the transfer was aborted by the client. The operation could not be completed as specified."}, {-375322, "LabVIEW: (Hex 0xFFFA45E6) IO processing is not active"}, {-375321, "LabVIEW: (Hex 0xFFFA45E7) There is not enough power to complete the requested operation."}, {-375320, "LabVIEW: (Hex 0xFFFA45E8) The requested resource has been removed."}, {-375319, "LabVIEW: (Hex 0xFFFA45E9) The supplied buffer is too small."}, {-375318, "LabVIEW: (Hex 0xFFFA45EA) A hardware failure has occurred. The operation could not be completed as specified."}, {-375317, "LabVIEW: (Hex 0xFFFA45EB) The operation you requested is redundant or invalid when the object is in this state."}, {-375316, "LabVIEW: (Hex 0xFFFA45EC) Thread was running when you attempted to start it (redundant state change)."}, {-375315, "LabVIEW: (Hex 0xFFFA45ED) The acquisition of the synchronization object failed"}, {-375314, "LabVIEW: (Hex 0xFFFA45EE) The synchronization object was abandoned by the previous holder"}, {-375313, "LabVIEW: (Hex 0xFFFA45EF) The name or handle requested has already been reserved by another client"}, {-375312, "LabVIEW: (Hex 0xFFFA45F0) There is no more data available to read or no more space available in which to write."}, {-375311, "LabVIEW: (Hex 0xFFFA45F1) The operation has begun and will complete asynchronously."}, {-375310, "LabVIEW: (Hex 0xFFFA45F2) The requested resource must be initialized before use."}, {-375309, "LabVIEW: (Hex 0xFFFA45F3) The requested resource has been marked for deletion and is rejecting new requests."}, {-375308, "LabVIEW: (Hex 0xFFFA45F4) An unexpected operationg system error occurred."}, {-375307, "LabVIEW: (Hex 0xFFFA45F5) The requested operation did not complete in time."}, {-375306, "LabVIEW: (Hex 0xFFFA45F6) The requested resource was not located."}, {-375305, "LabVIEW: (Hex 0xFFFA45F7) The user passed an invalid parameter."}, {-375304, "LabVIEW: (Hex 0xFFFA45F8) The dynamic cast operation failed."}, {-375303, "LabVIEW: (Hex 0xFFFA45F9) An unexpected software error occurred."}, {-375302, "LabVIEW: (Hex 0xFFFA45FA) The requested feature is not supported."}, {-375301, "LabVIEW: (Hex 0xFFFA45FB) The memory could not be page locked"}, {-375300, "LabVIEW: (Hex 0xFFFA45FC) The specified number of bytes could not be allocated."}, {-375201, "LabVIEW: (Hex 0xFFFA465F) There was an unexpected error during the current operation."}, {-375200, "LabVIEW: (Hex 0xFFFA4660) Not enough memory to complete current operation."}, {-375108, "LabVIEW: (Hex 0xFFFA46BC) Invalid certificate ID."}, {-375107, "LabVIEW: (Hex 0xFFFA46BD) Certificate storage is out of space."}, {-375106, "LabVIEW: (Hex 0xFFFA46BE) Invalid files posted."}, {-375105, "LabVIEW: (Hex 0xFFFA46BF) Incorrect password."}, {-375104, "LabVIEW: (Hex 0xFFFA46C0) Private key mismatch."}, {-375103, "LabVIEW: (Hex 0xFFFA46C1) Invalid private key file."}, {-375102, "LabVIEW: (Hex 0xFFFA46C2) Wrong certificate type."}, {-375101, "LabVIEW: (Hex 0xFFFA46C3) Invalid certificate file."}, {-375100, "LabVIEW: (Hex 0xFFFA46C4) Unexpected error."}, {-375012, "LabVIEW: (Hex 0xFFFA471C) A JSON numeric value is out of the range of a LabVIEW numeric type."}, {-375011, "LabVIEW: (Hex 0xFFFA471D) LabVIEW failed to read or write a -Infinity or +Infinity floating-point value. You must enable LabVIEW JSON extensions to allow support for a value of Infinity."}, {-375010, "LabVIEW: (Hex 0xFFFA471E) LabVIEW failed to read or write a NaN floating-point value. You must enable LabVIEW JSON extensions to allow support for a value of NaN."}, {-375009, "LabVIEW: (Hex 0xFFFA471F) The JSON string contains an invalid multi-dimensional array."}, {-375008, "LabVIEW: (Hex 0xFFFA4720) The array has an invalid number of dimensions."}, {-375007, "LabVIEW: (Hex 0xFFFA4721) The cluster or JSON string contains an invalid number of elements. When strict validation is enabled, the number of elements in the JSON string must match the number of elements in the input cluster."}, {-375006, "LabVIEW: (Hex 0xFFFA4722) The cluster element was not found in the JSON string."}, {-375005, "LabVIEW: (Hex 0xFFFA4723) Type mismatch between JSON and LabVIEW."}, {-375004, "LabVIEW: (Hex 0xFFFA4724) The path cannot be found in the JSON string."}, {-375003, "LabVIEW: (Hex 0xFFFA4725) The JSON string is invalid. JSON strings must be encoded in UTF-8 and must conform to the JSON grammar."}, {-375002, "LabVIEW: (Hex 0xFFFA4726) The cluster element name is invalid. Each element of the cluster must have either a unique name or no name, such as an empty string."}, {-375001, "LabVIEW: (Hex 0xFFFA4727) The JSON root container must be an array or cluster."}, {-375000, "LabVIEW: (Hex 0xFFFA4728) The data type cannot be converted to or from JSON. Supported data types include arrays and clusters of booleans, numerics, strings, and other arrays and clusters."}, {-356060, "LabVIEW: (Hex 0xFFFA9124) LabVIEW Web Services: An unexpected communication error has occurred with the remote target. This error typically occurs when the LabVIEW application on the remote target has crashed or restarted unexpectedly. Subsequent calls to this Web service will attempt to repair the communication error. However, the application may no longer be in a known good state."}, {-356010, "LabVIEW: (Hex 0xFFFA9156) LabVIEW Web Services: The specified property or method cannot be used over a network. Execute this property or method only on the local host."}, {-356005, "LabVIEW: (Hex 0xFFFA915B) LabVIEW Web Services: Cannot connect to the remote target or the connection is refused."}, {-356004, "LabVIEW: (Hex 0xFFFA915C) LabVIEW Web Services: LabVIEW cannot find the I/O Variable Remote Configuration Web Service on the remote target. This Web service is not installed or has not loaded."}, {-356002, "LabVIEW: (Hex 0xFFFA915E) LabVIEW Web Services: LabVIEW could not find the specified I/O variable on the remote target. The remote target may have crashed or it may be rebooting. Check the status of your remote target. Then close and reopen the VI on the local host that references the I/O variable."}, {-316999, "LabVIEW: (Hex 0xFFFB29B9) An unknown error occurred when calling an Interface for MATLAB(R). Contact NI for technical support."}, {-316998, "LabVIEW: (Hex 0xFFFB29BA) Failed to connect to MATLAB(R). Make sure that you installed and activated MATLAB on the machine and try running the VI again."}, {-316997, "LabVIEW: (Hex 0xFFFB29BB) An unknown error occurred when LabVIEW writes data to the MATLAB(R) workspace. Contact NI for technical support."}, {-316996, "LabVIEW: (Hex 0xFFFB29BC) Failed to get data from the MATLAB(R) workspace. The data type(s) you specify in the Interface for MATLAB document must match the data type(s) of the actual data returned from the MATLAB function or script."}, {-316995, "LabVIEW: (Hex 0xFFFB29BD) Failed to find the .m file specified in the Interface for MATLAB(R)."}, {-316994, "LabVIEW: (Hex 0xFFFB29BE) An error occurred when calling the MATLAB(R) script or function."}, {-316989, "LabVIEW: (Hex 0xFFFB29C3) An unknown error occurred when calling an Interface for MATLAB(R). Contact NI for technical support."}, {-316988, "LabVIEW: (Hex 0xFFFB29C4) Failed to write data to the MATLAB(R) workspace."}, {-316987, "LabVIEW: (Hex 0xFFFB29C5) Failed to get data from the MATLAB(R) workspace."}, {-316986, "LabVIEW: (Hex 0xFFFB29C6) An error occurred when calling the MATLAB(R) function or script. Make sure that the MATLAB function or script works in MATLAB."}, {-314352, "LabVIEW: (Hex 0xFFFB3410) You cannot read data from a writer endpoint or write data to a reader endpoint. Ensure that you have not wired a Write Single Element to Stream, Write Multiple Elements to Stream, or Flush Stream function to a Create Network Stream Reader Endpoint function. Conversely, ensure that you have not wired a Read Single Element from Stream or Read Multiple Elements from Stream function to a Create Network Stream Writer Endpoint function."}, {-314351, "LabVIEW: (Hex 0xFFFB3411) You must read or write elements of the same data type that you wired to the data type terminal of the Create Network Stream Reader Endpoint or Create Network Stream Writer Endpoint function."}, {-314350, "LabVIEW: (Hex 0xFFFB3412) Another application is already streaming data to an endpoint in the context you specified. If you specified a context name in the reader name or writer name terminal of the endpoint, you must specify an unused context name. If you did not specify a context name, you must specify an unused context name by entering an endpoint URL in the reader name or writer name terminal."}, {-314340, "LabVIEW: (Hex 0xFFFB341C) The local endpoint found the remote endpoint at the URL you specified, but the remote endpoint was trying to connect to a third endpoint. Ensure that corresponding endpoints each specify the URL of the other endpoint, or specify a URL with only one of the endpoints so the other endpoint accepts a connection from the first endpoint that connects to it."}, {-314335, "LabVIEW: (Hex 0xFFFB3421) The local endpoint was restarted because the computer that hosts the remote endpoint crashed, was rebooted, or experienced a hang."}, {-314320, "LabVIEW: (Hex 0xFFFB3430) LabVIEW could not create the remote endpoint because the computer that hosts the endpoint ran out of memory."}, {-314310, "LabVIEW: (Hex 0xFFFB343A) The remote endpoint has been destroyed."}, {-314305, "LabVIEW: (Hex 0xFFFB343F) The protocol version of the writer endpoint is not compatible with the protocol version of the reader endpoint. To transfer data between these endpoints, you must upgrade the version of LabVIEW that the older endpoint uses."}, {-314302, "LabVIEW: (Hex 0xFFFB3442) The remote endpoint is already connected to another endpoint. Each endpoint can connect to only one other endpoint at a time."}, {-314246, "LabVIEW: (Hex 0xFFFB347A) The remote and local endpoints are either both reader endpoints or both writer endpoints. You can prompt a connection between a reader and writer endpoint only ."}, {-314245, "LabVIEW: (Hex 0xFFFB347B) The data type 
